vi "Get Default Value.vi"(9 "Index/Build Array":bool, 10 "Ctrl Name":string, 11 "Controls Refs[]":refnum<vi>[](array[refnum])) -> (1 "Ctl Refnum":refnum<vi>, 2 "Found?":bool, 3 "DefVal":variant)   [LabVIEW 2021]
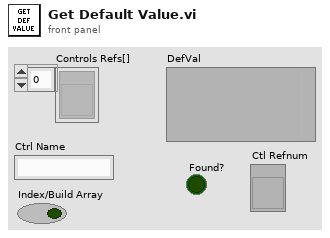
[diagram p1: front panel]
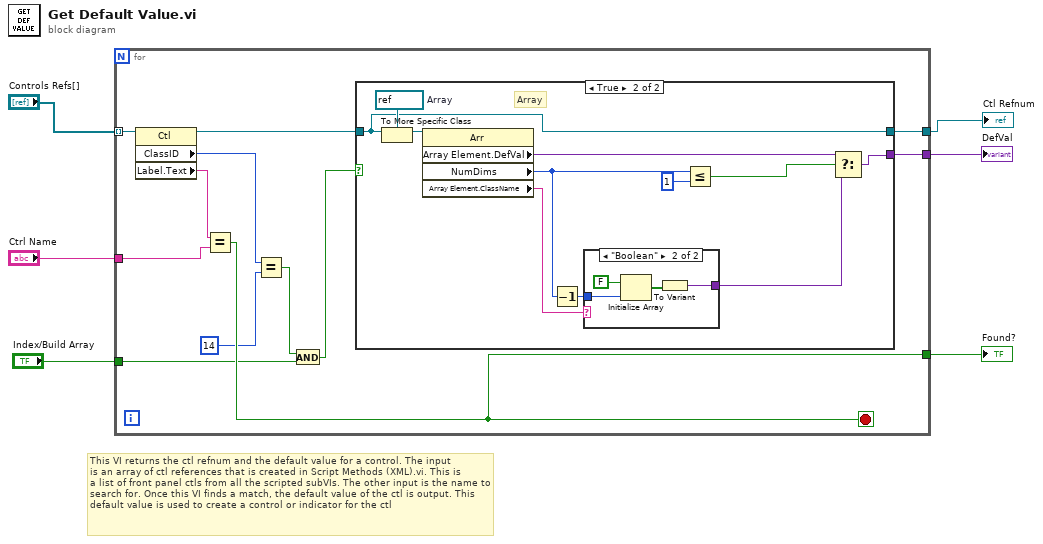
[diagram p0: block diagram]
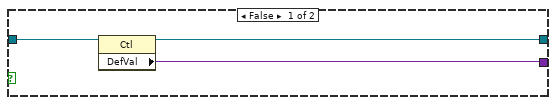
[diagram p2: hidden frame]
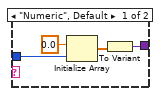
[diagram p3: hidden frame]
diagram:
  # "This VI returns the ctl refnum and the default value for a control. The input \nis an array of ctl references that is created in Script Methods (XML).vi. This is \na list of front panel ctls from all the scripted subVIs. The other input is the name to search for. Once this VI finds a match, the default value of the ctl is output. This default value is used to create a control or indicator for the ctl"
  n1 = for {
    tunnel: "Controls Refs[]" -> [w18] mode=indexing
    tunnel: "Ctrl Name" -> [w17]
    tunnel: [w14] -> w5
    tunnel: [w16] -> w6
    tunnel: [w13] -> w2
    tunnel: "Index/Build Array" -> [w9]
    stop <- w16 stop-if-true
    n2 = property class="Ctl"(reference=w18) -> (reference out=w15:refnum<vi>, "ClassID"=w8:u32, "Label.Text"=w12:string)  [unwired: 1 in, 1 out]
    n3 = Equal?(x=w12, y=w17) -> (x = y?=w16:bool)
    n4 = Equal?(x=w8, y=u32 14) -> (x = y?=w10:bool)
    n5 = And(x=w10, y=w9) -> (x .and. y?=w7:bool)
    n6 = case shown="True" w7 {
      tunnel: w15 -> [w21 w30]
      tunnel: [w19 w24] -> w14
      tunnel: [w20 w30] -> w13
      frame False {
        n7 = property class="Ctl"(reference=w21) -> (reference out=w20:refnum<vi>, "DefVal"=w19:variant)  [unwired: 1 in, 1 out]
      }
      frame True {
        w31 = refnum<vi> refnum  # Array
        # "Array"
        n8 = To More Specific Class(target class=w31, reference=w30) -> (specific class reference=w32:refnum<vi>)  [unwired: 1 in, 1 out]
        n9 = property class="Arr"(reference=w32) -> ("Array Element.DefVal"=w23:variant, "NumDims"=w26:u32, "Array Element.ClassName"=w27:string)  [unwired: 1 in, 2 out]
        n10 = Decrement(x=w26) -> (x-1=w25:u32)
        n11 = case shown="\"Boolean\"" w27 {
          tunnel: [w33 w37] -> w22
          tunnel: w25 -> [w35 w40]
          frame "Numeric", Default {
            n12 = Initialize Array(0.0, w35) -> (w34:dbl[])
            n13 = To Variant(anything=w34) -> (Variant=w33:variant)
          }
          frame "Boolean" {
            n14 = Initialize Array(FALSE, w40) -> (w38:bool[])
            n15 = To Variant(anything=w38) -> (Variant=w37:variant)
          }
        }
        n16 = Less Or Equal?(x=w26, y=u32 1) -> (x <= y?=w28:bool)
        n17 = Select(t=w23, s=w28, f=w22) -> (s? t:f=w24:variant)
      }
    }
  }
  "Found?" <- w6
  "DefVal" <- w5
  "Ctl Refnum" <- w2
